vi "Conversor C a F o F a C.vi"(1 "C o F":bool, 2 "Temperatura a convertir":dbl) -> (0 "Numeric":dbl)   [LabVIEW 2013]
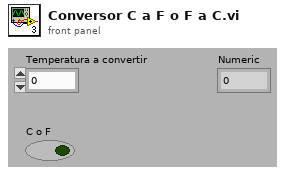
[diagram p1: front panel]
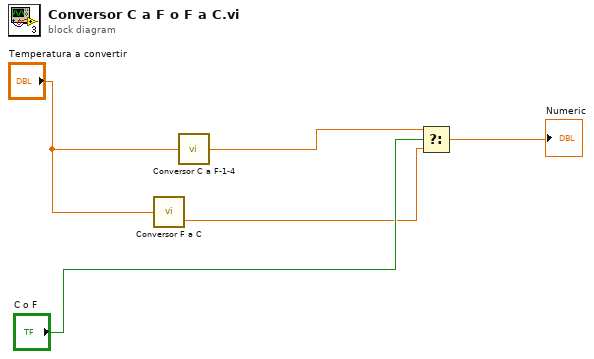
[diagram p0: block diagram]
diagram:
  n1 = call "Conversor F a C.vi"("Temperatura a convertir"="Temperatura a convertir") -> ("Temperatura convertida a F"=w3:dbl)  [unwired: 1 in]
  n2 = call "Conversor C a F-1-4.vi"("Temperatura a convertir"="Temperatura a convertir") -> ("Temp Convertida a C"=w1:dbl)
  n3 = Select(t=w1, s="C o F", f=w3) -> (s? t:f=→"Numeric":dbl)
